vi "Channel_FromClass.vi"(8 "error in (no error)":errorcluster, 10 "Channel.lvclass":refnum<class "Channel.lvclass">, 11 "Node Ptr":T1 format="%.0x") -> (0 "error out":errorcluster, 2 "Channel Ref":T1 format="%.0x", 3 "Node Ptr Out":T1 format="%.0x")   [LabVIEW 2024, in "Embedded TDMS Logger System Explorer.lvlib"]
doc: "Creates a channel in the VeriStand System Definition File Custom Device based on a Class definition of the Channel."
uses:
  Embedded TDMS Logger System Explorer.lvlib
  Shared/File Classes/Channel/Channel.lvclass
  <vilib>/NI VeriStand/Custom Device API/Custom Device Item Ref.ctl
  <vilib>/NI VeriStand/Custom Device API/Custom Device Channel.ctl
  <vilib>/NI VeriStand/Custom Device API/Custom Device Channel Type.ctl
  Shared/Constants.vi
  <vilib>/NI VeriStand/Custom Device API/Set Item Property (Dependent Node Pointer).vi
  <vilib>/NI VeriStand/Custom Device API/Set Item Property (I32).vi
  <vilib>/NI VeriStand/Custom Device API/Set Item Property (Variant).vi
  <vilib>/NI VeriStand/Custom Device API/Set Item Property (Boolean).vi
  <vilib>/NI VeriStand/Custom Device API/Custom Device API.lvlib
  Shared/Embedded TDMS Logger Shared.lvlib
  <vilib>/NI VeriStand/Custom Device Tools/Custom Device Utility Library/Custom Device Utility Library.lvlib
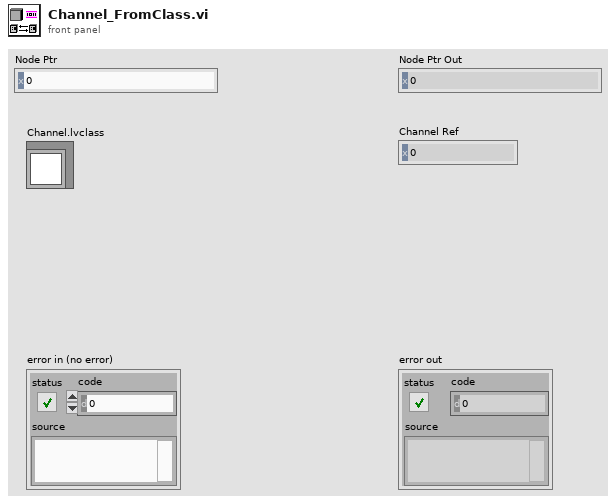
[diagram p1: front panel]
types:
  T1 = typedef "Custom Device API.lvlib/Custom Device Item Ref.ctl" = u64
  T2 = typedef "Custom Device API.lvlib/Custom Device Channel.ctl" = cluster{"Type":T3, "Units":string, "Default Value":dbl, "Faultable":bool, "Scalable":bool}
  T3 = typedef "Custom Device API.lvlib/Custom Device Channel Type.ctl" = enum16{"Input", "Output"}
  T4 = typedef "Meta Data.ctl" = cluster{"Key":string, "Value":string}
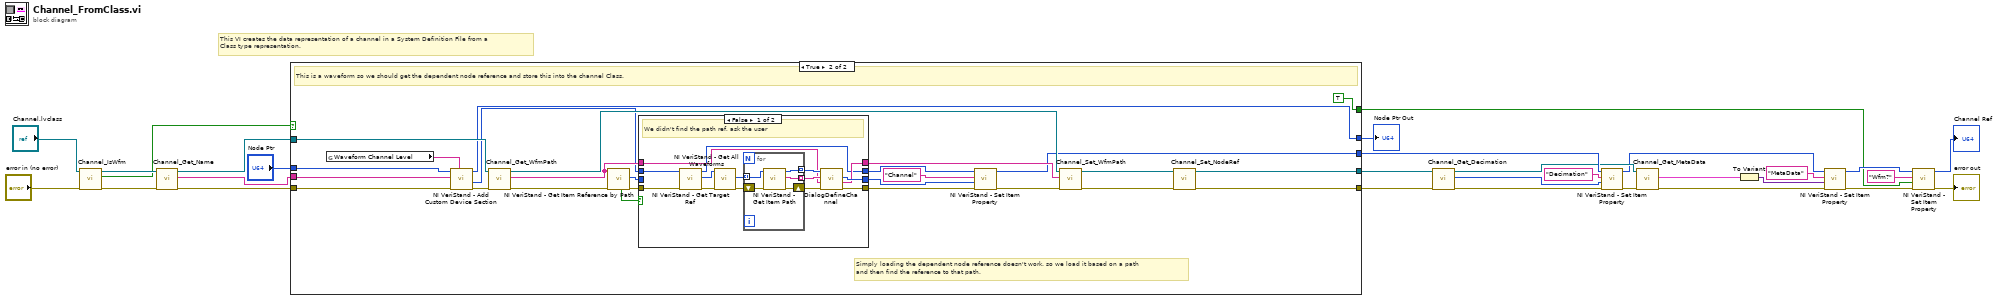
[diagram p0: block diagram]
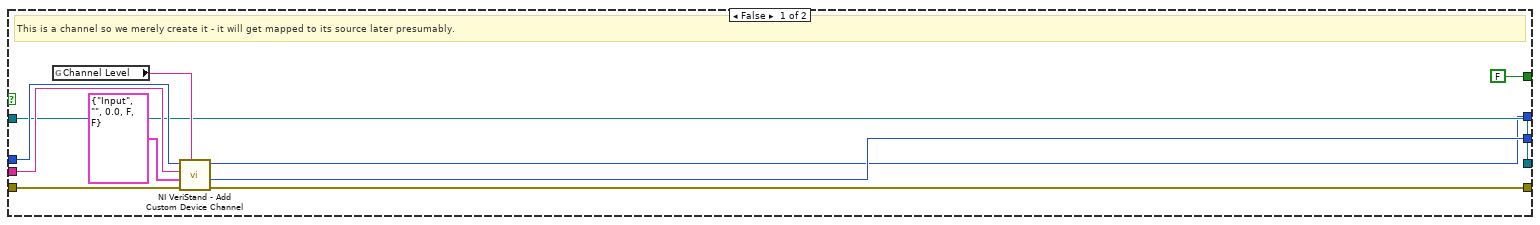
[diagram p2: hidden frame]
diagram:
  # "This VI creates the data representation of a channel in a System Definition File from a\nClass type representation."
  n1 = call-dynamic "Channel_IsWfm.vi"("error in (no error)"="error in (no error)", "Channel in"="Channel.lvclass") -> ("error out"=w27:errorcluster, "Wfm?"=w17:bool, "Channel out"=w25:refnum<class "Channel.lvclass">)  [unwired: 7 in]
  n2 = call-dynamic "Channel_Get_Name.vi"("error in (no error)"=w27, "Channel in"=w25) -> ("error out"=w26:errorcluster, "Name"=w24:string, "Channel out"=w9:refnum<class "Channel.lvclass">)  [unwired: 7 in]
  n3 = case shown="True" w17 {
    tunnel: "Node Ptr" -> [w39 w65]
    tunnel: w26 -> [w38 w64]
    tunnel: w24 -> [w37 w63]
    tunnel: [w33 w47] -> w15
    tunnel: [w34 w44] -> w14
    tunnel: w9 -> [w32 w49]
    tunnel: [w32 w48] -> w8
    tunnel: [w31 w43] -> w5
    tunnel: [FALSE TRUE] -> w1
    frame False {
      # "This is a channel so we merely create it - it will get mapped to its source later presumably."
      n4 = global read "Constants.vi" "Channel Level"() -> (w35:string)
      n5 = call <vilib>:"NI VeriStand - Add Custom Device Channel.vi"("GUID (Default Channel)"=w35, "error in (no error)"=w38, "Channel"=T2 {"Type"=enum."Input", "Units"="", "Default Value"=0.0, "Faultable"=FALSE, "Scalable"=FALSE}, "Channel Name"=w37, "Parent Ref in"=w39) -> ("error out"=w33:errorcluster, "Channel Ref"=w34:T1, "Parent Ref out"=w31:T1)  [unwired: 3 in, 1 out]
    }
    frame True {
      # "Simply loading the dependent node reference doesn't work. so we load it based on a path\nand then find the reference to that path."
      # "This is a waveform so we should get the dependent node reference and store this into the channel Class."
      n6 = global read "Constants.vi" "Waveform Channel Level"() -> (w62:string)
      n7 = call <vilib>:"NI VeriStand - Add Custom Device Section.vi"("GUID (Default Section)"=w62, "error in (no error)"=w64, "Section Name"=w63, "Parent Ref in"=w65) -> ("error out"=w50:errorcluster, "Section Ptr"=w42:T1, "Parent Ref out"=w43:T1)  [unwired: 3 in, 2 out]
      n8 = call-dynamic "Channel_Get_WfmPath.vi"("error in (no error)"=w50, "Channel in"=w49) -> ("error out"=w51:errorcluster, "WfmPath"=w55:string, "Channel out"=w52:refnum<class "Channel.lvclass">)  [unwired: 7 in]
      n9 = call <vilib>:"NI VeriStand - Get Item Reference by Path.vi"("error in (no error)"=w51, "Item Path in"=w55) -> ("error out"=w59:errorcluster, "Item Ref"=w57:T1, "Found"=w60:bool)  [unwired: 6 in, 1 out]
      n10 = case shown="False" w60 {
        tunnel: w59 -> [w70 w88]
        tunnel: [w79 w88] -> w58
        tunnel: [w78 w87] -> w56
        tunnel: w57 -> [_ w87]
        tunnel: w55 -> [w72 w86]
        tunnel: [w71 w86] -> w54
        tunnel: w42 -> [w67 w85]
        tunnel: [w66 w85] -> w41
        frame False {
          # "We didn't find the path ref, ask the user"
          n11 = call <vilib>:"NI VeriStand - Get Target Ref.vi"("error in"=w70, "Item Ref in"=w67) -> ("error out"=w69:errorcluster, "Target Ref"=w68:T1, "Item Ref out"=w66:T1)  [unwired: 6 in, 1 out]
          n12 = call <vilib>:"NI VeriStand - Get All Waveforms.vi"("error in"=w69, "Section Ref in"=w68) -> ("error out"=w76:errorcluster, "Waveform Refs"=w77:T1[])  [unwired: 6 in, 2 out]
          n13 = for {
            tunnel: w77 -> [w84] mode=indexing
            shift-right: [w82] -> w73
            shift-left: w76 -> [w83]
            tunnel: [w81] -> w75 mode=indexing
            tunnel: [w80] -> w74 mode=indexing
            n14 = call <vilib>:"NI VeriStand - Get Item Path.vi"("error in (no error)"=w83, "Item Ref in"=w84) -> ("error out"=w82:errorcluster, "Path"=w80:string, "Item Ref out"=w81:T1)  [unwired: 6 in, 1 out]
          }
          n15 = call "DialogDefineChannel.vi"("error in"=w73, "Input String"=w72, "Available Paths"=w74, "Available Refs"=w75) -> ("error out"=w79:errorcluster, "Selected Path"=w71:string, "Selected Ref"=w78:T1)  [unwired: 4 in, 1 out]
        }
        frame True {
        }
      }
      n16 = call-poly <vilib>:"NI VeriStand - Set Item Property.vi"("error in (no error)"=w58, "Dependent Node Ref"=w56, "Property Name"="Channel", "Item Ref in"=w41) -> ("error out"=w53:errorcluster, "Item Ref out"=w44:T1)  [unwired: 5 in, 1 out]
      n17 = call-dynamic "Channel_Set_WfmPath.vi"("error in (no error)"=w53, "WfmPath"=w54, "Channel in"=w52) -> ("error out"=w45:errorcluster, "Channel out"=w46:refnum<class "Channel.lvclass">)  [unwired: 7 in]
      n18 = call-dynamic "Channel_Set_NodeRef.vi"("error in (no error)"=w45, "Channel in"=w46) -> ("error out"=w47:errorcluster, "Channel out"=w48:refnum<class "Channel.lvclass">)  [unwired: 8 in]
    }
  }
  "Node Ptr Out" <- w5
  n19 = call-dynamic "Channel_Get_Decimation.vi"("error in (no error)"=w15, "Channel in"=w8) -> ("error out"=w16:errorcluster, "Decimation"=w11:i32, "Channel out"=w4:refnum<class "Channel.lvclass">)  [unwired: 7 in]
  n20 = call-poly <vilib>:"NI VeriStand - Set Item Property.vi"("error in (no error)"=w16, "Value"=w11, "Property Name"="Decimation", "Item Ref in"=w14) -> ("error out"=w3:errorcluster, "Item Ref out"=w2:T1)  [unwired: 5 in, 1 out]
  n21 = call-dynamic "Channel_Get_MetaData.vi"("error in (no error)"=w3, "Channel in"=w4) -> ("error out"=w12:errorcluster, "Meta Data"=w13:T4[])  [unwired: 7 in, 1 out]
  n22 = To Variant(anything=w13) -> (Variant=w23:variant)
  n23 = call-poly <vilib>:"NI VeriStand - Set Item Property.vi"("error in (no error)"=w12, "Value"=w23, "Property Name"="MetaData", "Item Ref in"=w2) -> ("error out"=w22:errorcluster, "Item Ref out"=w21:T1)  [unwired: 5 in, 1 out]
  n24 = call-poly <vilib>:"NI VeriStand - Set Item Property.vi"("error in (no error)"=w22, "Value"=w1, "Property Name"="Wfm?", "Item Ref in"=w21) -> ("error out"=→"error out":errorcluster, "Item Ref out"=→"Channel Ref":T1)  [unwired: 5 in, 1 out]
